vi "Func-엑셀 데이터를 그래프로 출력.vi"() -> ()   [LabVIEW 2015] (continued)
\n206.98\n206.99\n207.01\n207.03\n207.04\n207.06\n207.08\n207.09\n207.11\n207.13\n207.14\n207.16\n207.18\n207.19\n207.21\n207.23\n207.24\n207.26\n207.28\n207.3\n207.31\n207.33\n207.34\n207.36\n207.38\n207.4\n207.41\n207.43\n207.44\n207.46\n207.48\n207.49\n207.51\n207.53\n207.54\n207.56\n207.58\n207.59\n207.61\n207.63\n207.65\n207.66\n207.68\n207.69\n207.71\n207.73\n207.75\n207.76\n207.78\n207.79\n207.81\n207.83\n207.84\n207.86\n207.88\n207.89\n207.91\n207.93\n207.94\n207.96\n207.98\n207.99\n208.01\n208.03\n208.04\n208.06\n208.08\n208.09\n208.11\n208.13\n208.14\n208.16\n208.18\n208.19\n208.21\n208.23\n208.24\n208.26\n208.28\n208.29\n208.31\n208.33\n208.35\n208.36\n208.38\n208.39\n208.41\n208.43\n208.44\n208.46\n208.48\n208.49\n208.51\n208.53\n208.54\n208.56\n208.58\n208.6\n208.61\n208.63\n208.64\n208.66\n208.68\n208.69\n208.71\n208.73\n208.74\n208.76\n208.78\n208.79\n208.81\n208.83\n208.84\n208.86\n208.88\n208.9\n208.91\n208.93\n208.94\n208.96\n208.98\n208.99\n209.01\n209.03\n209.04\n209.06\n209.08\n209.09\n209.11\n209.13\n209.14\n209.16\n209.18\n209.19\n209.21\n209.23\n209.24\n209.26\n209.28\n209.29\n209.31\n209.33\n209.34\n209.36\n209.38\n209.39\n209.41\n209.43\n209.44\n209.46\n209.48\n209.49\n209.51\n209.53\n209.54\n209.56\n209.58\n209.59\n209.61\n209.63\n209.64\n209.66\n209.68\n209.69\n209.71\n209.73\n209.74\n209.76\n209.78\n209.79\n209.81\n209.83\n209.84\n209.86\n209.88\n209.89\n209.91\n209.93\n209.94\n209.96\n209.98\n209.99\n210.01\n210.03\n210.04\n210.06\n210.08\n210.09\n210.11\n210.13\n210.15\n210.16\n210.18\n210.19\n210.21\n210.23\n210.24\n210.26\n210.28\n210.29\n210.31\n210.33\n210.34\n210.36\n210.38\n210.4\n210.41\n210.43\n210.44\n210.46\n210.48\n210.5\n210.51\n210.53\n210.54\n210.56\n210.58\n210.59\n210.61\n210.63\n210.64\n210.66\n210.68\n210.69\n210.71\n210.73\n210.75\n210.76\n210.78\n210.79\n210.81\n210.83\n210.85\n210.86\n210.88\n210.89\n210.91\n210.93\n210.94\n210.96\n210.98\n210.99\n211.01\n211.03\n211.04\n211.06\n211.08\n211.09\n211.11\n211.13\n211.14\n211.16\n211.18\n211.2\n211.21\n211.23\n211.24\n211.26\n211.28\n211.29\n211.31\n211.33\n211.34\n211.36\n211.38\n211.39\n211.41\n211.43\n211.44\n211.46\n211.48\n211.49\n211.51\n211.53\n211.54\n211.56\n211.58\n211.59\n211.61\n211.63\n211.64\n211.66\n211.68\n211.69\n211.71\n211.73\n211.74\n211.76\n211.78\n211.79\n211.81\n211.83\n211.84\n211.86\n211.88\n211.89\n211.91\n211.93\n211.94\n211.96\n211.98\n211.99\n212.01\n212.03\n212.04\n212.06\n212.08\n212.09\n212.11\n212.13\n212.14\n212.16\n212.18\n212.19\n212.21\n212.23\n212.24\n212.26\n212.28\n212.29\n212.31\n212.33\n212.34\n212.36\n212.38\n212.39\n212.41\n212.43\n212.44\n212.46\n212.48\n212.49\n212.51\n212.53\n212.54\n212.56\n212.58\n212.59\n212.61\n212.63\n212.64\n212.66\n212.68\n212.69\n212.71\n212.73\n212.74\n212.76\n212.78\n212.79\n212.81\n212.83\n212.84\n212.86\n212.88\n212.89\n212.91\n212.93\n212.94\n212.96\n212.98\n212.99\n213.01\n213.03\n213.04\n213.06\n213.08\n213.09\n213.11\n213.13\n213.14\n213.16\n213.18\n213.19\n213.21\n213.23\n213.24\n213.26\n213.28\n213.29\n213.31\n213.33\n213.34\n213.36\n213.38\n213.39\n213.41\n213.43\n213.44\n213.46\n213.48\n213.5\n213.51\n213.53\n213.54\n213.56\n213.58\n213.59\n213.61\n213.63\n213.64\n213.66\n213.68\n213.69\n213.71\n213.73\n213.74\n213.76\n213.78\n213.79\n213.81\n213.83\n213.85\n213.86\n213.88\n213.89\n213.91\n213.93\n213.95\n213.96\n213.98\n213.99\n214.01\n214.03\n214.04\n214.06\n214.08\n214.09\n214.11\n214.13\n214.14\n214.16\n214.18\n214.2\n214.21\n214.23\n214.24\n214.26\n214.28\n214.29\n214.31\n214.33\n214.34\n214.36\n214.38\n214.39\n214.41\n214.43\n214.44\n214.46\n214.48\n214.49\n214.51\n214.53\n214.54\n214.56\n214.58\n214.59\n214.61\n214.63\n214.64\n214.66\n214.68\n214.69\n214.71\n214.73\n214.74\n214.76\n214.78\n214.8\n214.81\n214.83\n214.84\n214.86\n214.88\n214.9\n214.91\n214.93\n214.94\n214.96\n214.98\n214.99\n215.01\n215.03\n215.04\n215.06\n215.08\n215.09\n215.11\n215.13\n215.14\n215.16\n215.18\n215.19\n215.21\n215.23\n215.24\n215.26\n215.28\n215.29\n215.31\n215.33\n215.34\n215.36\n215.38\n215.39\n215.41\n215.43\n215.44\n215.46\n215.48\n215.49\n215.51\n215.53\n215.54\n215.56\n215.58\n215.59\n215.61\n215.63\n215.64\n215.66\n215.68\n215.69\n215.71\n215.73\n215.74\n215.76\n215.78\n215.79\n215.81\n215.83\n215.84\n215.86\n215.88\n215.89\n215.91\n215.93\n215.94\n215.96\n215.98\n215.99\n216.01\n216.03\n216.04\n216.06\n216.08\n216.09\n216.11\n216.13\n216.14\n216.16\n216.18\n216.19\n216.21\n216.23\n216.24\n216.26\n216.28\n216.29\n216.31\n216.33\n216.34\n216.36\n216.38\n216.39\n216.41\n216.43\n216.44\n216.46\n216.48\n216.49\n216.51\n216.53\n216.54\n216.56\n216.58\n216.6\n216.61\n216.63\n216.64\n216.66\n216.68\n216.69\n216.71\n216.73\n216.74\n216.76\n216.78\n216.79\n216.81\n216.83\n216.84\n216.86\n216.88\n216.89\n216.91\n216.93\n216.95\n216.96\n216.98\n216.99\n217.01\n217.03\n217.05\n217.06\n217.08\n217.09\n217.11\n217.13\n217.14\n217.16\n217.18\n217.19\n217.21\n217.23\n217.24\n217.26\n217.28\n217.3\n217.31\n217.33\n217.34\n217.36\n217.38\n217.4\n217.41\n217.43\n217.44\n217.46\n217.48\n217.49\n217.51\n217.53\n217.54\n217.56\n217.58\n217.59\n217.61\n217.63\n217.65\n217.66\n217.68\n217.69\n217.71\n217.73\n217.74\n217.76\n217.78\n217.79\n217.81\n217.83\n217.84\n217.86\n217.88\n217.89\n217.91\n217.93\n217.94\n217.96\n217.98\n217.99\n218.01\n218.03\n218.04\n218.06\n218.08\n218.09\n218.11\n218.13\n218.14\n218.16\n218.18\n218.19\n218.21\n218.23\n218.24\n218.26\n218.28\n218.29\n218.31\n218.33\n218.34\n218.36\n218.38\n218.39\n218.41\n218.43\n218.44\n218.46\n218.48\n218.49\n218.51\n218.53\n218.54\n218.56\n218.58\n218.59\n218.61\n218.63\n218.64\n218.66\n218.68\n218.69\n218.71\n218.73\n218.74\n218.76\n218.78\n218.79\n218.81\n218.83\n218.84\n218.86\n218.88\n218.89\n218.91\n218.93\n218.94\n218.96\n218.98\n218.99\n219.01\n219.03\n219.04\n219.06\n219.08\n219.09\n219.11\n219.13\n219.14\n219.16\n219.18\n219.19\n219.21\n219.23\n219.24\n219.26\n219.28\n219.29\n219.31\n219.33\n219.34\n219.36\n219.38\n219.39\n219.41\n219.43\n219.44\n219.46\n219.48\n219.49\n219.51\n219.53\n219.54\n219.56\n219.58\n219.59\n219.61\n219.63\n219.64\n219.66\n219.68\n219.7\n219.71\n219.73\n219.74\n219.76\n219.78\n219.8\n219.81\n219.83\n219.84\n219.86\n219.88\n219.89\n219.91\n219.93\n219.94\n219.96\n219.98\n219.99\n220.01\n220.03\n220.05\n220.06\n220.08\n220.09\n220.11\n220.13\n220.15\n220.16\n220.18\n220.19\n220.21\n220.23\n220.24\n220.26\n220.28\n220.29\n220.31\n220.33\n220.34\n220.36\n220.38\n220.4\n220.41\n220.43\n220.44\n220.46\n220.48\n220.49\n220.51\n220.53\n220.54\n220.56\n220.58\n220.59\n220.61\n220.63\n220.65\n220.66\n220.68\n220.69\n220.71\n220.73\n220.74\n220.76\n220.78\n220.79\n220.81\n220.83\n220.84\n220.86\n220.88\n220.89\n220.91\n220.93\n220.94\n220.96\n220.98\n221\n221.01\n221.03\n221.04\n221.06\n221.08\n221.09\n221.11\n221.13\n221.14\n221.16\n221.18\n221.2\n221.21\n221.23\n221.24\n221.26\n221.28\n221.29\n221.31\n221.33\n221.34\n221.36\n221.38\n221.39\n221.41\n221.43\n221.44\n221.46\n221.48\n221.49\n221.51\n221.53\n221.54\n221.56\n221.58\n221.59\n221.61\n221.63\n221.64\n221.66\n221.68\n221.69\n221.71\n221.73\n221.74\n221.76\n221.78\n221.79\n221.81\n221.83\n221.84\n221.86\n221.88\n221.89\n221.91\n221.93\n221.94\n221.96\n221.98\n221.99\n222.01\n222.03\n222.04\n222.06\n222.08\n222.09\n222.11\n222.13\n222.14\n222.16\n222.18\n222.19\n222.21\n222.23\n222.24\n222.26\n222.28\n222.29\n222.31\n222.33\n222.34\n222.36\n222.38\n222.39\n222.41\n222.43\n222.44\n222.46\n222.48\n222.49\n222.51\n222.53\n222.54\n222.56\n222.58\n222.59\n222.61\n222.63\n222.64\n222.66\n222.68\n222.69\n222.71\n222.73\n222.74\n222.76\n222.78\n222.79\n222.81\n222.83\n222.84\n222.86\n222.88\n222.9\n222.91\n222.93\n222.94\n222.96\n222.98\n222.99\n223.01\n223.03\n223.04\n223.06\n223.08\n223.09\n223.11\n223.13\n223.15\n223.16\n223.18\n223.19\n223.21\n223.23\n223.25\n223.26\n223.28\n223.29\n223.31\n223.33\n223.34\n223.36\n223.38\n223.4\n223.41\n223.43\n223.44\n223.46\n223.48\n223.49\n223.51\n223.53\n223.54\n223.56\n223.58\n223.59\n223.61\n223.63\n223.64\n223.66\n223.68\n223.69\n223.71\n223.73\n223.74\n223.76\n223.78\n223.79\n223.81\n223.83\n223.84\n223.86\n223.88\n223.89\n223.91\n223.93\n223.94\n223.96\n223.98\n223.99\n224.01\n224.03\n224.04\n224.06\n224.08\n224.09\n224.11\n224.13\n224.14\n224.16\n224.18\n224.19\n224.21\n224.23\n224.24\n224.26\n224.28\n224.29\n224.31\n224.33\n224.34\n224.36\n224.38\n224.39\n224.41\n224.43\n224.44\n224.46\n224.48\n224.49\n224.51\n224.53\n224.54\n224.56\n224.58\n224.59\n224.61\n224.63\n224.64\n224.66\n224.68\n224.69\n224.71\n224.73\n224.74\n224.76\n224.78\n224.79\n224.81\n224.83\n224.84\n224.86\n224.88\n224.89\n224.91\n224.93\n224.94\n224.96\n224.98\n224.99\n225.01\n225.03\n225.04\n225.06\n225.08\n225.09\n225.11\n225.13\n225.14\n225.16\n225.18\n225.19\n225.21\n225.23\n225.24\n225.26\n225.28\n225.29\n225.31\n225.33\n225.34\n225.36\n225.38\n225.39\n225.41\n225.43\n225.44\n225.46\n225.48\n225.49\n225.51\n225.53\n225.54\n225.56\n225.58\n225.59\n225.61\n225.63\n225.64\n225.66\n225.68\n225.69\n225.71\n225.73\n225.74\n225.76\n225.78\n225.79\n225.81\n225.83\n225.84\n225.86\n225.88\n225.9\n225.91\n225.93\n225.94\n225.96\n225.98\n226\n226.01\n226.03\n226.04\n226.06\n226.08\n226.09\n226.11\n226.13\n226.14\n226.16\n226.18\n226.19\n226.21\n226.23\n226.25\n226.26\n226.28\n226.29\n226.31\n226.33\n226.35\n226.36\n226.38\n226.39\n226.41\n226.43\n226.44\n226.46\n226.48\n226.49\n226.51\n226.53\n226.54\n226.56\n226.58\n226.6\n226.61\n226.63\n226.64\n226.66\n226.68\n226.69\n226.71\n226.73\n226.74\n226.76\n226.78\n226.79\n226.81\n226.83\n226.85\n226.86\n226.88\n226.89\n226.91\n226.93\n226.95\n226.96\n226.98\n226.99\n227.01\n227.03\n227.04\n227.06\n227.08\n227.09\n227.11\n227.13\n227.14\n227.16\n227.18\n227.19\n227.21\n227.23\n227.24\n227.26\n227.28\n227.29\n227.31\n227.33\n227.34\n227.36\n227.38\n227.39\n227.41\n227.43\n227.44\n227.46\n227.48\n227.49\n227.51\n227.53\n227.54\n227.56\n227.58\n227.59\n227.61\n227.63\n227.64\n227.66\n227.68\n227.69\n227.71\n227.73\n227.74\n227.76\n227.78\n227.79\n227.81\n227.83\n227.84\n227.86\n227.88\n227.89\n227.91\n227.93\n227.94\n227.96\n227.98\n227.99\n228.01\n228.03\n228.04\n228.06\n228.08\n228.09\n228.11\n228.13\n228.14\n228.16\n228.18\n228.19\n228.21\n228.23\n228.24\n228.26\n228.28\n228.29\n228.31\n228.33\n228.34\n228.36\n228.38\n228.39\n228.41\n228.43\n228.44\n228.46\n228.48\n228.49\n228.51\n228.53\n228.54\n228.56\n228.58\n228.59\n228.61\n228.63\n228.64\n228.66\n228.68\n228.69\n228.71\n228.73\n228.75\n228.76\n228.78\n228.79\n228.81\n228.83\n228.84\n228.86\n228.88\n228.89\n228.91\n228.93\n228.94\n228.96\n228.98\n229\n229.01\n229.03\n229.04\n229.06\n229.08\n229.1\n229.11\n229.13\n229.14\n229.16\n229.18\n229.19\n229.21\n229.23\n229.24\n229.26\n229.28\n229.29\n229.31\n229.33\n229.35\n229.36\n229.38\n229.39\n229.41\n229.43\n229.45\n229.46\n229.48\n229.49\n229.51\n229.53\n229.54\n229.56\n229.58\n229.59\n229.61\n229.63\n229.64\n229.66\n229.68\n229.7\n229.71\n229.73\n229.74\n229.76\n229.78\n229.79\n229.81\n229.83\n229.84\n229.86\n229.88\n229.89\n229.91\n229.93\n229.94\n229.96\n229.98\n229.99\n230.01\n230.03\n230.04\n230.06\n230.08\n230.09\n230.11\n230.13\n230.14\n230.16\n230.18\n230.19\n230.21\n230.23\n230.25\n230.26\n230.28\n230.29\n230.31\n230.33\n230.34\n230.36\n230.38\n230.39\n230.41\n230.43\n230.44\n230.46\n230.48\n230.5\n230.51\n230.53\n230.54\n230.56\n230.58\n230.59\n230.61\n230.63\n230.64\n230.66\n230.68\n230.69\n230.71\n230.73\n230.74\n230.76\n230.78\n230.79\n230.81\n230.83\n230.84\n230.86\n230.88\n230.89\n230.91\n230.93\n230.94\n230.96\n230.98\n230.99\n231.01\n231.03\n231.04\n231.06\n231.08\n231.09\n231.11\n231.13\n231.14\n231.16\n231.18\n231.19\n231.21\n231.23\n231.24\n231.26\n231.28\n231.29\n231.31\n231.33\n231.34\n231.36\n231.38\n231.39\n231.41\n231.43\n231.44\n231.46\n231.48\n231.49\n231.51\n231.53\n231.54\n231.56\n231.58\n231.59\n231.61\n231.63\n231.64\n231.66\n231.68\n231.69\n231.71\n231.73\n231.74\n231.76\n231.78\n231.79\n231.81\n231.83\n231.84\n231.86\n231.88\n231.89\n231.91\n231.93\n231.94\n231.96\n231.98\n231.99\n232.01\n232.03\n232.04\n232.06\n232.08\n232.1\n232.11\n232.13\n232.14\n232.16\n232.18\n232.19\n232.21\n232.23\n232.24\n232.26\n232.28\n232.29\n232.31\n232.33\n232.34\n232.36\n232.38\n232.39\n232.41\n232.43\n232.45\n232.46\n232.48\n232.49\n232.51\n232.53\n232.55\n232.56\n232.58\n232.59\n232.61\n232.63\n232.64\n232.66\n232.68\n232.69\n232.71\n232.73\n232.74\n232.76\n232.78\n232.79\n232.81\n232.83\n232.84\n232.86\n232.88\n232.9\n232.91\n232.93\n232.94\n232.96\n232.98\n233\n233.01\n233.03\n233.04\n233.06\n233.08\n233.09\n233.11\n233.13\n233.14\n233.16\n233.18\n233.19\n233.21\n233.23\n233.24\n233.26\n233.28\n233.29\n233.31\n233.33\n233.35\n233.36\n233.38\n233.39\n233.41\n233.43\n233.44\n233.46\n233.48\n233.49\n233.51\n233.53\n233.54\n233.56\n233.58\n233.59\n233.61\n233.63\n233.64\n233.66\n233.68\n233.69\n233.71\n233.73\n233.74\n233.76\n233.78\n233.79\n233.81\n233.83\n233.84\n233.86\n233.88\n233.89\n233.91\n233.93\n233.94\n233.96\n233.98\n233.99\n234.01\n234.03\n234.04\n234.06\n234.08\n234.09\n234.11\n234.13\n234.14\n234.16\n234.18\n234.19\n234.21\n234.23\n234.24\n234.26\n234.28\n234.29\n234.31\n234.33\n234.34\n234.36\n234.38\n234.39\n234.41\n234.43\n234.44\n234.46\n234.48\n234.49\n234.51\n234.53\n234.54\n234.56\n234.58\n234.59\n234.61\n234.63\n234.64\n234.66\n234.68\n234.69\n234.71\n234.73\n234.74\n234.76\n234.78\n234.79\n234.81\n234.83\n234.84\n234.86\n234.88\n234.89\n234.91\n234.93\n234.94\n234.96\n234.98\n234.99\n235.01\n235.03\n235.04\n235.06\n235.08\n235.09\n235.11\n235.13\n235.14\n235.16\n235.18\n235.2\n235.21\n235.23\n235.24\n235.26\n235.28\n235.29\n235.31\n235.33\n235.34\n235.36\n235.38\n235.39\n235.41\n235.43\n235.44\n235.46\n235.48\n235.49\n235.51\n235.53\n235.55\n235.56\n235.58\n235.59\n235.61\n235.63\n235.65\n235.66\n235.68\n235.69\n235.71\n235.73\n235.74\n235.76\n235.78\n235.79\n235.81\n235.83\n235.84\n235.86\n235.88\n235.9\n235.91\n235.93\n235.94\n235.96\n235.98\n236\n236.01\n236.03\n236.04\n236.06\n236.08\n236.09\n236.11\n236.13\n236.14\n236.16\n236.18\n236.19\n236.21\n236.23\n236.24\n236.26\n236.28\n236.29\n236.31\n236.33\n236.34\n236.36\n236.38\n236.39\n236.41\n236.43\n236.44\n236.46\n236.48\n236.49\n236.51\n236.53\n236.54\n236.56\n236.58\n236.6\n236.61\n236.63\n236.64\n236.66\n236.68\n236.69\n236.71\n236.73\n236.75\n236.76\n236.78\n236.79\n236.81\n236.83\n236.84\n236.86\n236.88\n236.89\n236.91\n236.93\n236.94\n236.96\n236.98\n236.99\n237.01\n237.03\n237.04\n237.06\n237.08\n237.09\n237.11\n237.13\n237.14\n237.16\n237.18\n237.19\n237.21\n237.23\n237.24\n237.26\n237.28\n237.29\n237.31\n237.33\n237.34\n237.36\n237.38\n237.39\n237.41\n237.43\n237.44\n237.46\n237.48\n237.49\n237.51\n237.53\n237.54\n237.56\n237.58\n237.59\n237.61\n237.63\n237.64\n237.66\n237.68\n237.69\n237.71\n237.73\n237.74\n237.76\n237.78\n237.79\n237.81\n237.83\n237.84\n237.86\n237.88\n237.89\n237.91\n237.93\n237.94\n237.96\n237.98\n237.99\n238.01\n238.03\n238.04\n238.06\n238.08\n238.09\n238.11\n238.13\n238.14\n238.16\n238.18\n238.19\n238.21\n238.23\n238.24\n238.26\n238.28\n238.29\n238.31\n238.33\n238.34\n238.36\n238.38\n238.4\n238.41\n238.43\n238.44\n238.46\n238.48\n238.49\n238.51\n238.53\n238.54\n238.56\n238.58\n238.59\n238.61\n238.63\n238.65\n238.66\n238.68\n238.69\n238.71\n238.73\n238.75\n238.76\n238.78\n238.79\n238.81\n238.83\n238.84\n238.86\n238.88\n238.89\n238.91\n238.93\n238.94\n238.96\n238.98\n239\n239.01\n239.03\n239.04\n239.06\n239.08\n239.09\n239.11\n239.13\n239.14\n239.16\n239.18\n239.19\n239.21\n239.23\n239.25\n239.26\n239.28\n239.29\n239.31\n239.33\n239.35\n239.36\n239.38\n239.39\n239.41\n239.43\n239.44\n239.46\n239.48\n239.49\n239.51\n239.53\n239.54\n239.56\n239.58\n239.59\n239.61\n239.63\n239.64\n239.66\n239.68\n239.69\n239.71\n239.73\n239.74\n239.76\n239.78\n239.79\n239.81\n239.83\n239.84\n239.86\n239.88\n239.89\n239.91\n239.93\n239.94\n239.96\n239.98\n239.99\n240.01\n240.03\n240.04\n240.06\n240.08\n240.09\n240.11\n240.13\n240.14\n240.16\n240.18\n240.19\n240.21\n240.23\n240.24\n240.26\n240.28\n240.29\n240.31\n240.33\n240.34\n240.36\n240.38\n240.39\n240.41\n240.43\n240.44\n240.46\n240.48\n240.49\n240.51\n240.53\n240.54\n240.56\n240.58\n240.59\n240.61\n240.63\n240.64\n240.66\n240.68\n240.69\n240.71\n240.73\n240.74\n240.76\n240.78\n240.79\n240.81\n240.83\n240.84\n240.86\n240.88\n240.89\n240.91\n240.93\n240.94\n240.96\n240.98\n240.99\n241.01\n241.03\n241.04\n241.06\n241.08\n241.09\n241.11\n241.13\n241.14\n241.16\n241.18\n241.19\n241.21\n241.23\n241.24\n241.26\n241.28\n241.29\n241.31\n241.33\n241.34\n241.36\n241.38\n241.39\n241.41\n241.43\n241.44\n241.46\n241.48\n241.5\n241.51\n241.53\n241.54\n241.56\n241.58\n241.59\n241.61\n241.63\n241.64\n241.66\n241.68\n241.69\n241.71\n241.73\n241.75\n241.76\n241.78\n241.79\n241.81\n241.83\n241.85\n241.86\n241.88\n241.89\n241.91\n241.93\n241.94\n241.96\n241.98\n241.99\n242.01\n242.03\n242.04\n242.06\n242.08\n242.1\n242.11\n242.13\n242.14\n242.16\n242.18\n242.2\n242.21\n242.23\n242.24\n242.26\n242.28\n242.29\n242.31\n242.33\n242.34\n242.36\n242.38\n242.39\n242.41\n242.43\n242.45\n242.46\n242.48\n242.49\n242.51\n242.53\n242.54\n242.56\n242.58\n242.59\n258.82\n258.99\n259.16\n259.32\n259.49\n259.66\n259.82\n259.99\n260.16\n260.32\n260.49\n260.66\n260.83\n261\n261.16\n261.33\n261.5\n261.66\n261.83\n262\n262.16\n262.33\n262.51\n262.67\n262.84\n263.01\n263.17\n263.34\n263.51\n263.67\n263.84\n264.01\n264.17\n264.34\n264.51\n264.67\n264.84\n265.01\n265.17\n265.34\n265.51\n265.67\n265.84\n266.01\n266.17\n266.34\n266.51\n266.67\n266.84\n267.01\n267.17\n267.34\n267.51\n267.67\n267.84\n268.01\n268.17\n268.34\n268.51\n268.67\n268.84\n269.01\n269.17\n269.35\n269.51\n269.68\n269.85\n270.02\n270.18\n270.35\n270.51\n270.68\n270.85\n271.01\n271.18\n271.35\n271.51\n271.68\n271.85\n272.01\n272.18\n272.35\n272.52\n272.68\n272.85\n273.02\n273.18\n273.35\n273.51\n273.69\n273.86\n274.02\n274.19\n274.36\n274.52\n274.69\n274.86\n275.02\n275.19\n275.36\n275.52\n275.69\n275.86\n276.02\n276.19\n276.36\n276.52\n276.69\n276.86\n277.02\n277.19\n277.36\n277.52\n277.69\n277.86\n278.02\n278.19\n278.36\n278.52\n278.69\n278.86\n279.02\n279.19\n279.36\n279.52\n279.69\n279.86\n280.02\n280.19\n280.36\n280.52\n280.69\n280.86\n281.02\n281.19\n281.36\n281.52\n281.69\n281.86\n282.02\n282.19\n282.36\n282.52\n282.69\n282.86\n283.02\n283.19\n283.36\n283.52\n283.69\n283.86\n284.02\n284.19\n284.36\n284.52\n284.69\n284.86\n285.02\n285.19\n285.36\n285.52\n285.69\n285.86\n286.02\n286.19\n286.36\n286.52\n286.69\n286.86\n287.02\n287.19\n287.36\n287.52\n287.69\n287.86\n288.02\n288.19\n288.36\n288.52\n288.69\n288.86\n289.02\n289.19\n289.36\n289.52\n289.69\n289.86\n290.02\n290.19\n290.36\n290.53\n290.7\n290.86\n291.03\n291.2\n291.37\n291.53\n291.7\n291.86\n292.03\n292.2\n292.36\n292.53\n292.7\n292.86\n293.03\n293.2\n293.36\n293.53\n293.7\n293.87\n294.03\n294.2\n294.36\n294.53\n294.7\n294.86\n295.03\n295.2\n295.36\n295.53\n295.7\n295.86\n296.03\n296.2\n296.36\n296.53\n296.7\n296.87\n297.03\n297.2\n297.36\n297.53\n297.7\n297.86\n298.03\n298.2\n298.36\n298.53\n298.7\n298.86\n299.03\n299.2\n299.36\n299.53\n299.7\n299.86\n300.03\n300.2\n300.36\n300.53\n300.7\n300.86\n301.03\n301.2\n301.36\n301.53\n301.7\n301.86\n302.02\n302.03\n302.04\n302.06\n302.08\n302.09\n302.11\n302.13\n302.14\n302.16\n302.18\n302.19\n302.21\n302.23\n302.24\n302.26\n302.28\n302.29\n302.31\n302.33\n302.34\n302.36\n302.38\n302.39\n302.41\n302.43\n302.44\n302.46\n302.48\n302.49\n302.51\n302.53\n302.54\n302.56\n302.58\n302.59\n302.61\n302.63\n302.64\n302.66\n302.68\n302.69\n302.71\n302.73\n302.74\n302.76\n302.78\n302.8\n302.81\n302.83\n302.84\n302.86\n302.88\n302.89\n302.91\n302.93\n302.94\n302.96\n302.98\n302.99\n303.01\n303.03\n303.05\n303.06\n303.08\n303.09\n303.11\n303.13\n303.15\n303.16\n303.18\n303.19\n303.21\n303.23\n303.24\n303.26\n303.28\n303.29\n303.31\n303.33\n303.34\n303.36\n303.38\n303.4\n303.41\n303.43\n303.44\n303.46\n303.48\n303.5\n303.51\n303.53\n303.54\n303.56\n303.58\n303.59\n303.61\n303.63\n303.64\n303.66\n303.68\n303.69\n303.71\n303.73\n303.74\n303.76\n303.78\n303.79\n303.81\n303.83\n303.84\n303.86\n303.88\n303.89\n
